vi "打开离线文件.vi"() -> (0 "错误输出":errorcluster, 3 "文件句柄":i32)   [LabVIEW 2011]
uses:
  dll/em9636.dll
panel:
  out "文件路径":string
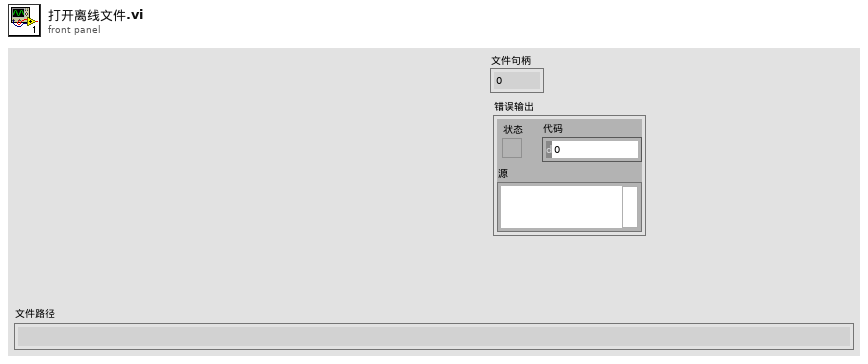
[diagram p1: front panel]
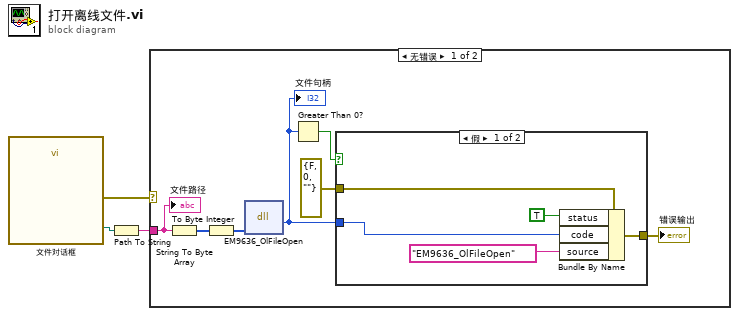
[diagram p0: block diagram]
diagram:
  n1 = call "文件对话框"() -> ("selected path"=w2:path, "error out"=w3:errorcluster)  [unwired: 12 in, 2 out]
  n2 = Path To String(path=w2) -> (string=w1:string)
  n3 = case shown="无错误" w3 {
    tunnel: w1 -> [w4 _]
    frame No Error {
      n4 = String To Byte Array(string=w4) -> (unsigned byte array=w10:u8[])
      n5 = To Byte Integer(number=w10) -> (8bit integer=w9:i8[])
      n6 = dll-call lib="PTH1abs Eèµ éç LABVIEWæºVI(v2.0)EM9636BD)EM9636BDè°ç¨APIå½æ°æ¹æ³éè®¯ä¾ç¨EM9636_demo_labview2011dll\nem9636.dll" fn="EM9636_OlFileOpen"("文件路径"=w9) -> ("文件句柄"=w5:i32)  [unwired: 4 in, 2 out]
      "文件句柄" <- w5
      n7 = Greater Than 0?(x=w5) -> (x > 0?=w8:bool)
      n8 = case shown="假" w8 {
        tunnel: [w13 w16] -> w7
        tunnel: errorcluster {"status"=FALSE, "code"=0, "source"=""} ("错误输出") -> [w15 w16]
        tunnel: w5 -> [w12 _]
        frame False {
          n9 = Bundle By Name(cluster=w15, "status"=TRUE, "code"=w12, "source"="EM9636_OlFileOpen") -> (w13:errorcluster)
        }
        frame True {
        }
      }
      "错误输出" <- w7
      "文件路径" <- w4
    }
    frame Error {
    }
  }
